vi "MarkerTactic.vi"(8 "error in (no error)":errorcluster, 9 "Game in":refnum<class "Game.lvclass">, 10 "Robot":refnum<class "Robot.lvclass">, 11 "MarkerTactic in":refnum<class "MarkerTactic.lvclass">) -> (0 "error out":errorcluster, 2 "Robot out":refnum<class "Robot.lvclass">, 3 "MarkerTactic out":refnum<class "MarkerTactic.lvclass">)   [LabVIEW 2018, in "MarkerTactic.lvclass"]
uses:
  MarkerTactic.lvclass
  C:/Users/lucas/Documents/RoboIME/SSL_AI - defense/Tactic_class/Tactic.lvclass
  Robot_class/Robot.lvclass
  Game_class/Game.lvclass
  Tactic_class/Tactic.lvclass/Tactic.ctl
  Game_class/Game.lvclass/Game.ctl
  Parameters_class/Parameters.lvclass/Parameters.ctl
  Skillbook_class/Skillbook.lvclass/Skillbook.ctl
  MarkerTactic.lvclass/MarkerTactic.ctl
  Skillbook_class/Read MarkerSkill.lvclass.vi
  Game_class/Read Parameters.lvclass.vi
  Parameters_class/Read Type of Marker.vi
  Tactic_class/Read Skillbook.vi
  Write States.vi
  Parameters_class/Parameters.lvclass
  Skillbook_class/Skillbook.lvclass
  MarkerSkill_class/MarkerSkill.lvclass
panel:
  out "x .or. y?":bool
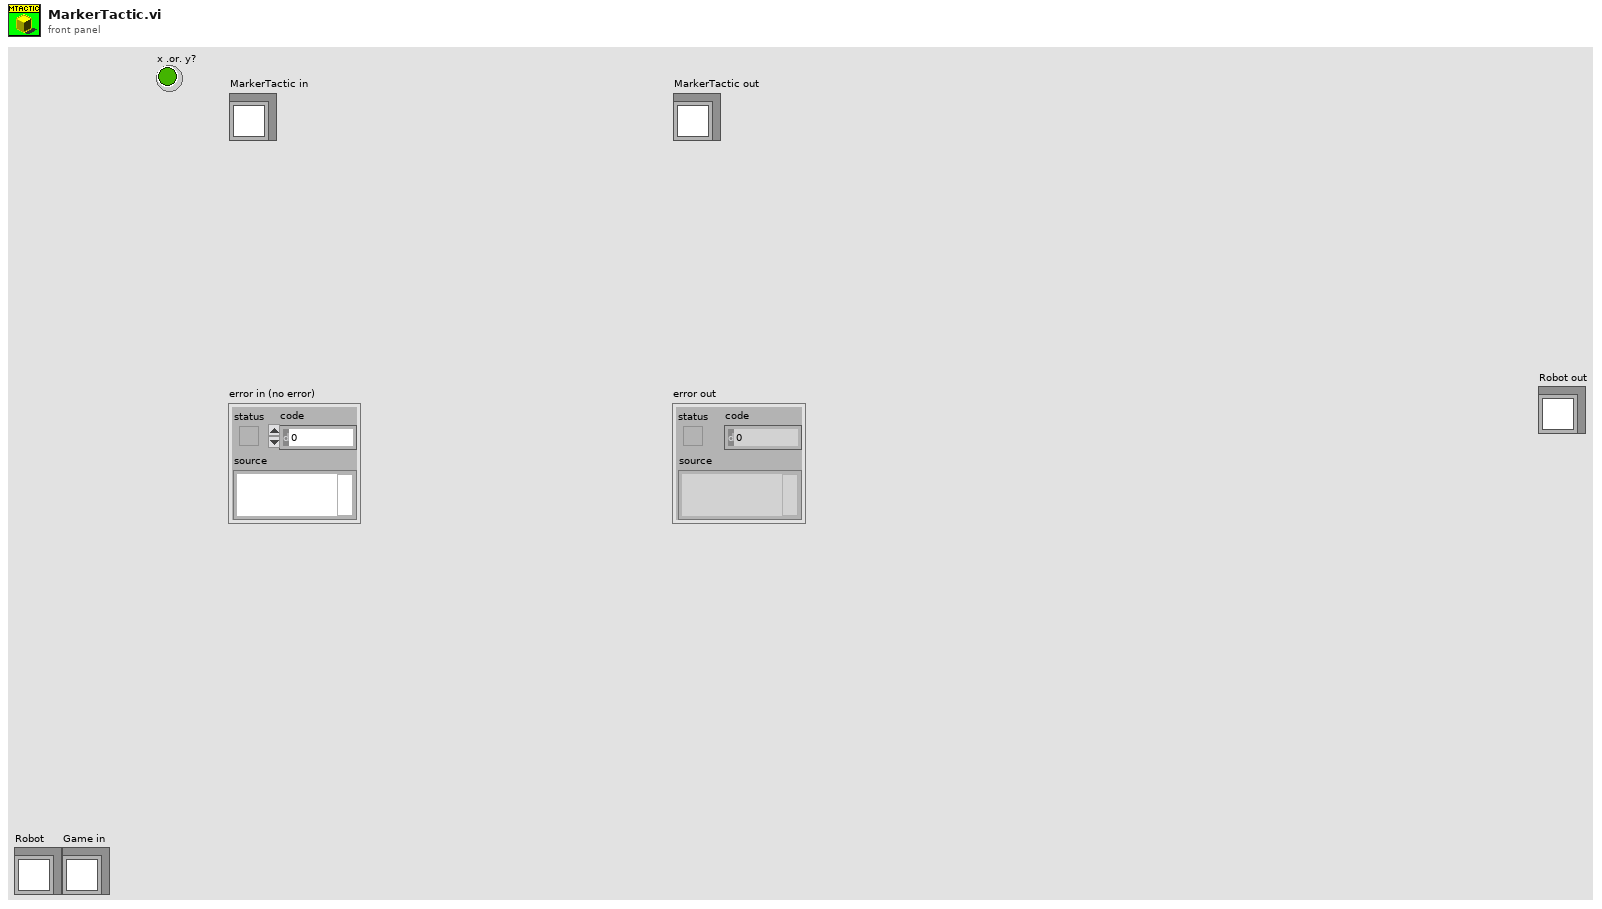
[diagram p1: front panel]
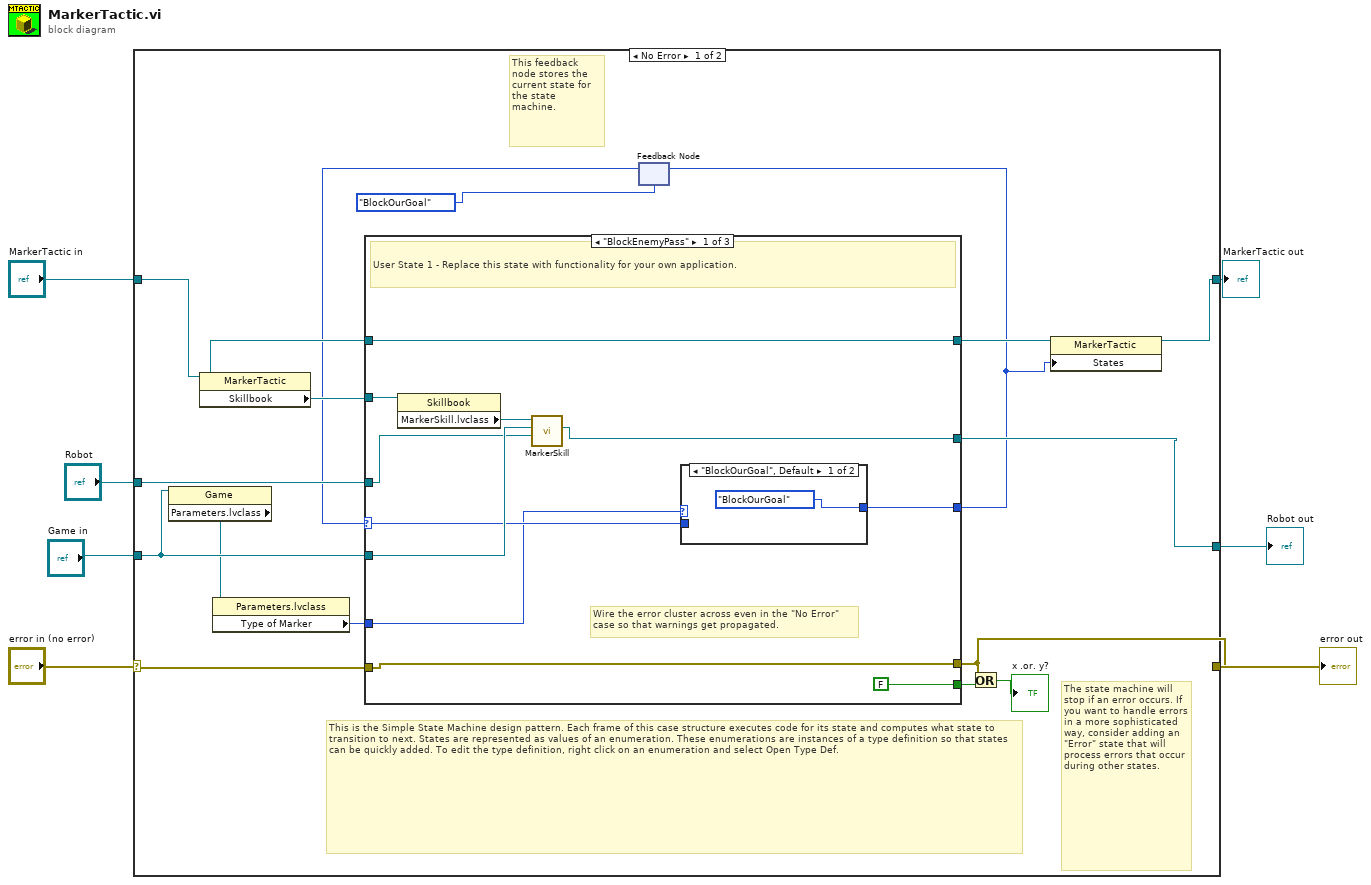
[diagram p0: block diagram]
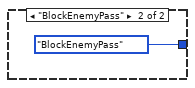
[diagram p2: hidden frame]
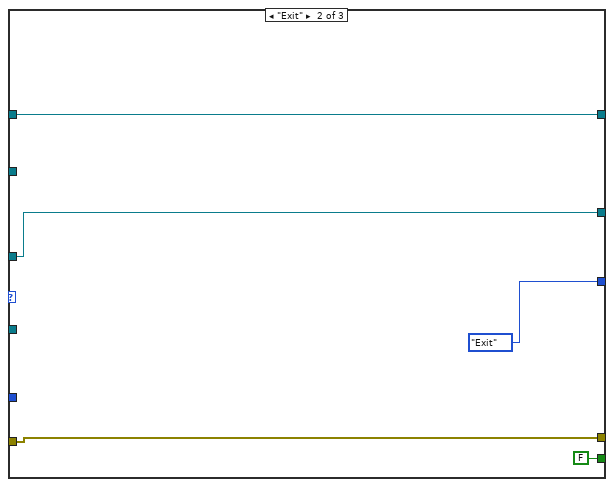
[diagram p3: hidden frame]
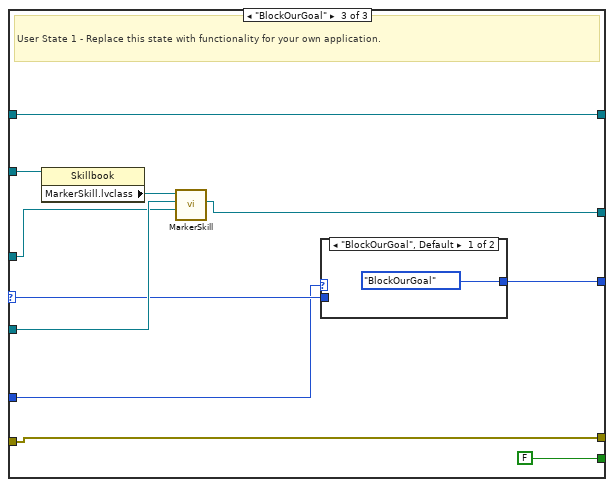
[diagram p4: hidden frame]
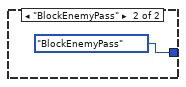
[diagram p5: hidden frame]
diagram:
  n1 = case shown="No Error" "error in (no error)" {
    selector: "error in (no error)" -> [w18 w57]
    tunnel: [w17 w57] -> w6
    tunnel: [w15 w56] -> w4
    tunnel: "MarkerTactic in" -> [w16 w56]
    tunnel: "Robot" -> [w19 w55]
    tunnel: "Game in" -> [w13 _]
    tunnel: [w14 w55] -> w1
    frame No Error {
      # "The state machine will stop if an error occurs. If you want to handle errors in a more sophisticated way, consider adding an \"Error\" state that will process errors that occur during other states."
      # "This feedback node stores the current state for the state machine."
      # "This is the Simple State Machine design pattern. Each frame of this case structure executes code for its state and computes what state to transition to next. States are represented as values of an enumeration. These enumerations are instances of a type definition so that states can be quickly added. To edit the type definition, right click on an enumeration and select Open Type Def."
      # "Wire the error cluster across even in the \"No Error\"\ncase so that warnings get propagated."
      n2 = property class="Game"(reference=w13) -> ("Parameters.lvclass"=w12:refnum<class "Parameters.lvclass">)  [unwired: 1 in, 2 out]
      n3 = property class="MarkerTactic"(reference=w16) -> ("Skillbook"=w21:refnum<class "Skillbook.lvclass">)  [unwired: 1 in, 2 out]
      n4 = property class="Parameters.lvclass"(reference=w12) -> ("Type of Marker"=w11:enum16{"BlockEnemyPass", "BlockOurGoal"})  [unwired: 1 in, 2 out]
      n5 = feedback #1(enum16{"Exit", "BlockOurGoal", "BlockEnemyPass"}."BlockOurGoal" ("States")) -> (w9:enum16{"Exit", "BlockOurGoal", "BlockEnemyPass"})
      n6 = case shown="\"BlockEnemyPass\"" w9 {
        selector: w9 -> [w25 _ w43]
        tunnel: [FALSE ("Stop Loop?") FALSE ("Stop Loop?") FALSE ("Stop Loop?")] -> w23
        tunnel: w21 -> [w33 _ w51]
        tunnel: w19 -> [w28 w39 w46]
        tunnel: [w27 w39 w45] -> w14
        tunnel: [w32 w40 w50] -> w20
        tunnel: w16 -> [w32 w40 w50]
        tunnel: w13 -> [w30 _ w48]
        tunnel: [w29 w38 w47] -> w17
        tunnel: w18 -> [w29 w38 w47]
        tunnel: [w26 enum16{"Exit", "BlockOurGoal", "BlockEnemyPass"}."Exit" ("States") w44] -> w8
        tunnel: w11 -> [w24 _ w42]
        frame "BlockEnemyPass" {
          # "User State 1 - Replace this state with functionality for your own application."
          n7 = property class="Skillbook"(reference=w33) -> ("MarkerSkill.lvclass"=w31:refnum<class "MarkerSkill.lvclass">)  [unwired: 1 in, 2 out]
          n8 = call-dynamic "MarkerSkill.vi"("Robot"=w28, "Game"=w30, "MarkerSkill in"=w31) -> ("Robot out"=w27:refnum<class "Robot.lvclass">)  [unwired: 6 in, 2 out]
          n9 = case shown="\"BlockOurGoal\", Default" w24 {
            tunnel: [enum16{"Exit", "BlockOurGoal", "BlockEnemyPass"}."BlockOurGoal" ("States") enum16{"Exit", "BlockOurGoal", "BlockEnemyPass"}."BlockEnemyPass" ("States")] -> w26
            tunnel: w25 -> [_ _]
            frame "BlockOurGoal", Default {
            }
            frame "BlockEnemyPass" {
            }
          }
        }
        frame "Exit" {
        }
        frame "BlockOurGoal" {
          # "User State 1 - Replace this state with functionality for your own application."
          n10 = property class="Skillbook"(reference=w51) -> ("MarkerSkill.lvclass"=w49:refnum<class "MarkerSkill.lvclass">)  [unwired: 1 in, 2 out]
          n11 = call-dynamic "MarkerSkill.vi"("Robot"=w46, "Game"=w48, "MarkerSkill in"=w49) -> ("Robot out"=w45:refnum<class "Robot.lvclass">)  [unwired: 6 in, 2 out]
          n12 = case shown="\"BlockOurGoal\", Default" w42 {
            tunnel: [enum16{"Exit", "BlockOurGoal", "BlockEnemyPass"}."BlockOurGoal" ("States") enum16{"Exit", "BlockOurGoal", "BlockEnemyPass"}."BlockEnemyPass" ("States")] -> w44
            tunnel: w43 -> [_ _]
            frame "BlockOurGoal", Default {
            }
            frame "BlockEnemyPass" {
            }
          }
        }
      }
      n13 = feedback-in #1(w8) -> ()
      n14 = Or(x=w17, y=w23) -> (x .or. y?=→"x .or. y?":bool)
      n15 = property class="MarkerTactic"(reference=w20, "States"=w8) -> (reference out=w15:refnum<class "MarkerTactic.lvclass">)  [unwired: 1 in, 1 out]
    }
    frame Error {
    }
  }
  "error out" <- w6
  "MarkerTactic out" <- w4
  "Robot out" <- w1
